vi "Get Delay.vi"(8 "error in (no error)":errorcluster, 10 "Channel (T0)":T1 items=["T0", "T1", "A", "B", "C", "D", "E", "F", "G", "H"], 11 "VISA resource name":refnum<visa-resource-name>) -> (0 "error out":errorcluster, 1 "Delay [s]":dbl format="%#_12g", 2 "relative to":T1 items=["T0", "T1", "A", "B", "C", "D", "E", "F", "G", "H"], 3 "VISA resource name out":refnum<visa-resource-name>, 4 "Device Errors":cluster{"code":i32, "Text":string}[](array[cluster]))   [LabVIEW 2014, in "Stanford Research DG645 - Driver.lvlib"]
doc: "Delay and Output Command: DLAY? c\nInstrument Error Check\n\nQuery the delay (in seconds) for channel c relative to another channel."
uses:
  Stanford Research DG645 - Driver.lvlib
  Channel.ctl
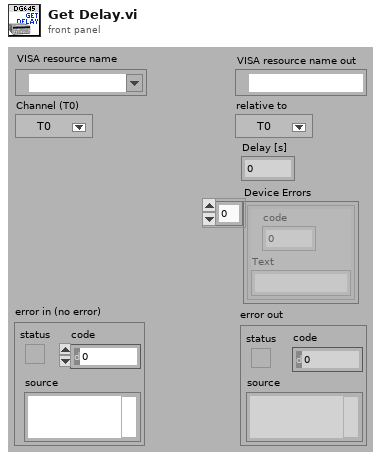
[diagram p1: front panel]
types:
  T1 = typedef "Stanford Research DG645 - Driver.lvlib/Channel.ctl" = i32
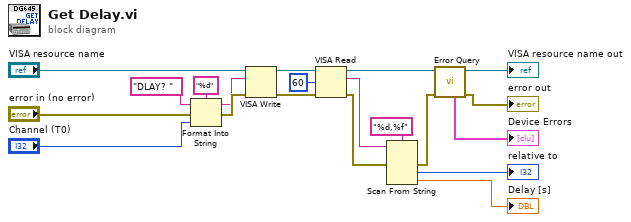
[diagram p0: block diagram]
diagram:
  n1 = Format Into String(format string="%d", initial string="DLAY? " ("command"), error in="error in (no error)", "Channel (T0)") -> (resulting string=w16:string, error out=w17:errorcluster)
  n2 = VISA Write(VISA resource name="VISA resource name", write buffer=w16, error in (no error)=w17) -> (VISA resource name out=w13:refnum<visa-resource-name>, error out=w12:errorcluster)  [unwired: 1 out]
  n3 = VISA Read(VISA resource name=w13, byte count=u32 60, error in (no error)=w12) -> (VISA resource name out=w11:refnum<visa-resource-name>, read buffer=w8:string, error out=w3:errorcluster)  [unwired: 1 out]
  n4 = Scan From String(format string="%d,%f", input string=w8, error in=w3) -> (error out=w2:errorcluster, output 1=→"relative to":T1, output 2=→"Delay [s]":dbl)  [unwired: 3 in, 2 out]
  n5 = call "Error Query.vi"("error in (no error)"=w2, "VISA resource name"=w11) -> ("error out"=→"error out":errorcluster, "VISA resource name out"=→"VISA resource name out":refnum<visa-resource-name>, "Device Errors"=→"Device Errors":cluster{"code":i32, "Text":string}[])  [unwired: 7 in]
